vi "XML Script - Move Diagram Code.vi"(8 "y":i16, 9 "x":i16, 11 "BlockDiagram XML":string) -> (3 "BlockDiagram XML out":string)   [LabVIEW 2017]
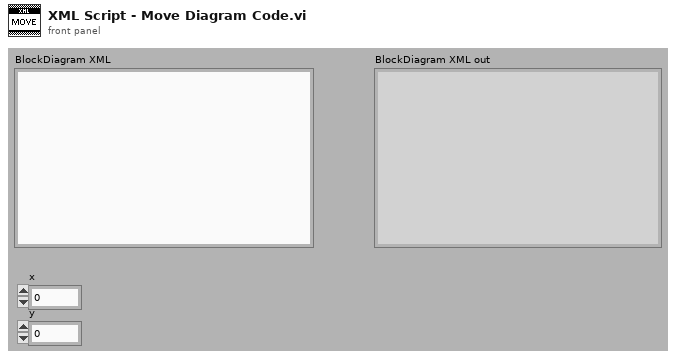
[diagram p1: front panel]
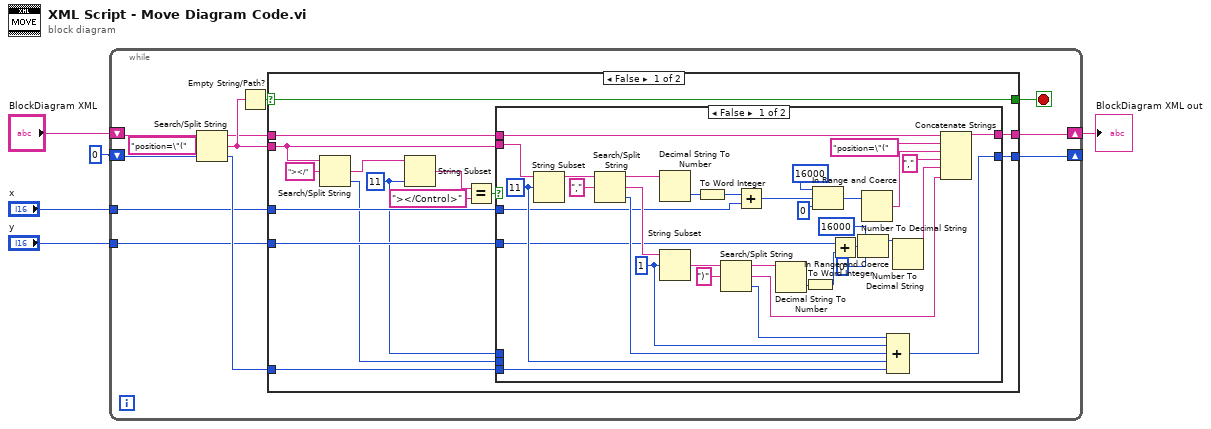
[diagram p0: block diagram]
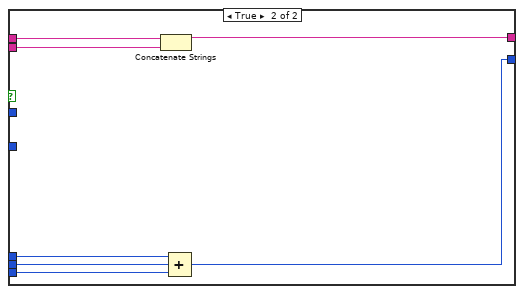
[diagram p2: hidden frame]
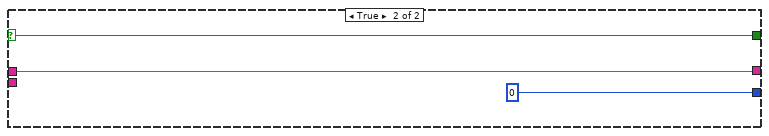
[diagram p3: hidden frame]
diagram:
  n1 = while {
    shift-right: [w13] -> _
    shift-left: 0 ("offset of match") -> [w6]
    shift-right: [w11] -> w5
    shift-left: "BlockDiagram XML" -> [w7]
    tunnel: "x" -> [w9]
    tunnel: "y" -> [w8]
    stop <- w12 stop-if-true
    n2 = Search/Split String(string=w7, search string/char (-)="position=\"(", offset (0)=w6) -> (substring before match=w15:string, match + rest of string=w16:string, offset of match=w10:i32)
    n3 = Empty String/Path?(string/path=w16) -> (empty?=w17:bool)
    n4 = case shown="False" w17 {
      selector: w17 -> [w31 w75]
      tunnel: w16 -> [w25 _]
      tunnel: w15 -> [w26 w77]
      tunnel: [w32 w77] -> w11
      tunnel: [w30 0 ("offset of match")] -> w13
      tunnel: [w31 w75] -> w12
      tunnel: w10 -> [w29 _]
      tunnel: w9 -> [w28 _]
      tunnel: w8 -> [w27 _]
      frame False {
        w18 = 11 ("offset (0)")
        n5 = Search/Split String(string=w25, search string/char (-)="></") -> (match + rest of string=w20:string, offset of match=w23:i32)  [unwired: 1 in, 1 out]
        n6 = String Subset(string=w20, length (rest)=w18) -> (substring=w19:string)  [unwired: 1 in]
        n7 = Equal?(x=w19, y="></Control>") -> (x = y?=w22:bool)
        n8 = case shown="False" w22 {
          tunnel: w26 -> [w61 w73]
          tunnel: w25 -> [w60 w74]
          tunnel: [w53 w72] -> w32
          tunnel: [w51 w70] -> w30
          tunnel: w29 -> [w47 w69]
          tunnel: w28 -> [w46 _]
          tunnel: w27 -> [w45 _]
          tunnel: w23 -> [_ w68]
          tunnel: w18 -> [_ w71]
          frame False {
            w48 = 11 ("offset (0)")
            w50 = 1 ("offset (0)")
            n9 = String Subset(string=w60, offset (0)=w48) -> (substring=w58:string)  [unwired: 1 in]
            n10 = Search/Split String(string=w58, search string/char (-)=",") -> (substring before match=w66:string, match + rest of string=w65:string, offset of match=w49:i32)  [unwired: 1 in]
            n11 = Decimal String To Number(string=w66) -> (number=w43:i32)  [unwired: 2 in, 1 out]
            n12 = String Subset(string=w65, offset (0)=w50) -> (substring=w64:string)  [unwired: 1 in]
            n13 = To Word Integer(number=w43) -> (16bit integer=w44:i16)
            n14 = Search/Split String(string=w64, search string/char (-)=")") -> (substring before match=w62:string, match + rest of string=w55:string, offset of match=w52:i32)  [unwired: 1 in]
            n15 = Add(x=w44, y=w46) -> (x+y=w40:i16)
            n16 = Decimal String To Number(string=w62) -> (number=w42:i32)  [unwired: 2 in, 1 out]
            n17 = To Word Integer(number=w42) -> (16bit integer=w41:i16)
            n18 = In Range and Coerce(upper limit=i16 16000, x=w40, lower limit=i16 0) -> (coerced(x)=w39:i16)  [unwired: 1 out]
            n19 = Add(x=w45, y=w41) -> (x+y=w36:i16)
            n20 = In Range and Coerce(upper limit=i16 16000, x=w36, lower limit=i16 0) -> (coerced(x)=w34:i16)  [unwired: 1 out]
            n21 = Number To Decimal String(number=w39) -> (decimal integer string=w57:string)  [unwired: 1 in]
            n22 = Compound Arithmetic op=ADD(w52, w50, w49, w48, w47) -> (w51:i32)
            n23 = Number To Decimal String(number=w34) -> (decimal integer string=w54:string)  [unwired: 1 in]
            n24 = Concatenate Strings(w61, "position=\"(" ("search string/char (-)"), w57, "," ("string"), w54, w55) -> (w53:string)
          }
          frame True {
            n25 = Concatenate Strings(w73, w74) -> (w72:string)
            n26 = Compound Arithmetic op=ADD(w71, w68, w69) -> (w70:i32)
          }
        }
      }
      frame True {
      }
    }
  }
  "BlockDiagram XML out" <- w5
